vi "Test myTree.vi"() -> ()   [LabVIEW 2015, in "MyTreeAPI.lvclass"]
uses:
  MyTreeAPI.lvclass
  Menubar/Menu.lvclass
panel:
  in  "Tree":string(tree)
  out "ItemTag":string
  out "Node ID":string
  in  "Tag":string
  in  "OK Button":bool
  in  "stop":bool
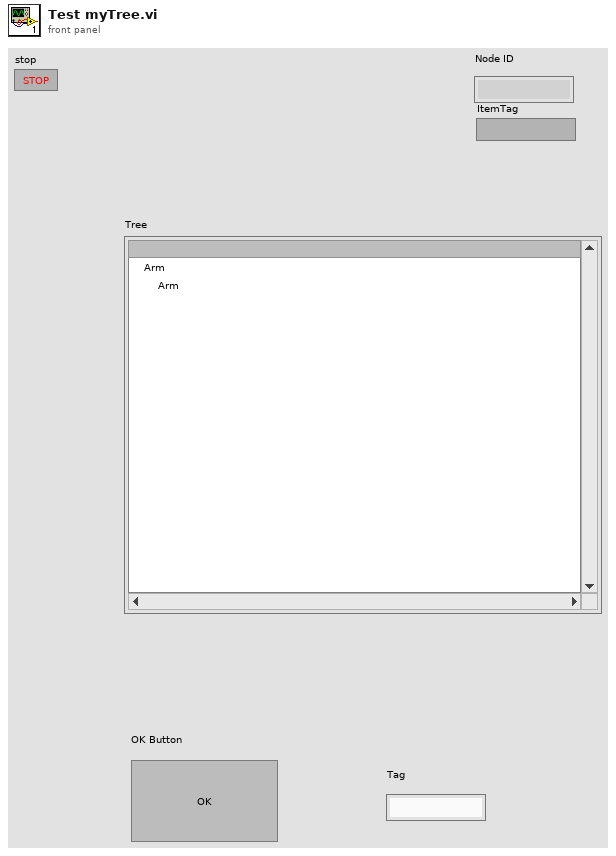
[diagram p1: front panel]
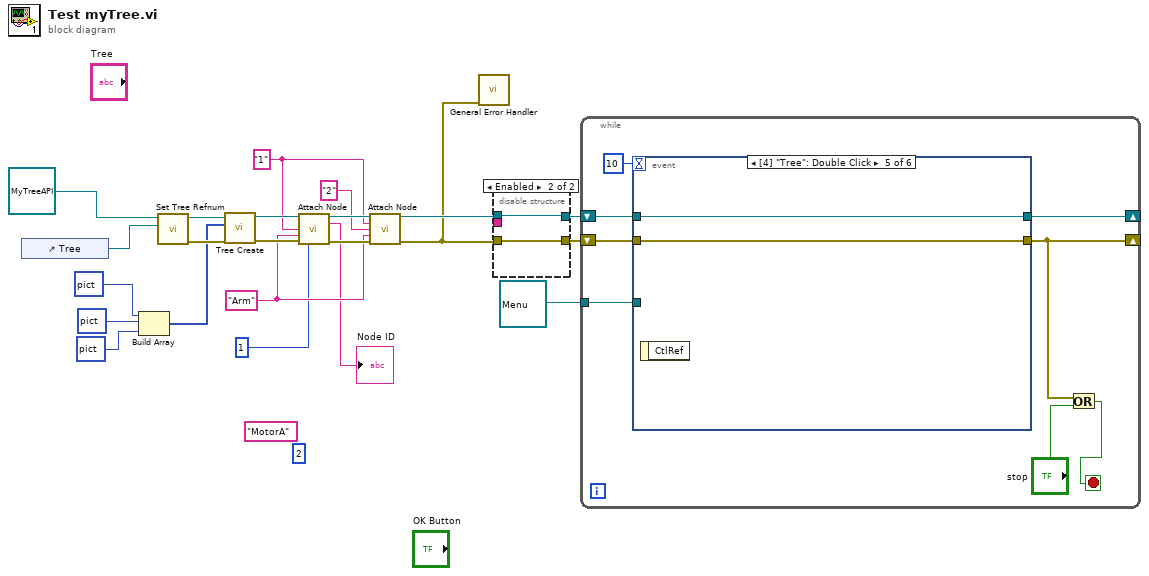
[diagram p0: block diagram]
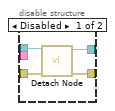
[diagram p2: hidden frame]
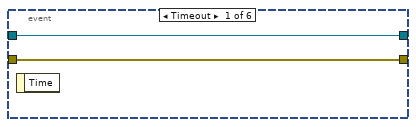
[diagram p3: hidden frame]
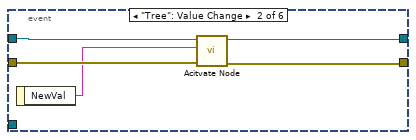
[diagram p4: hidden frame]
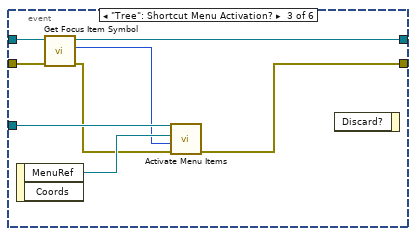
[diagram p5: hidden frame]
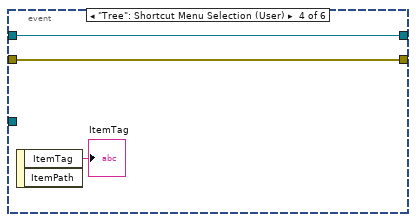
[diagram p6: hidden frame]
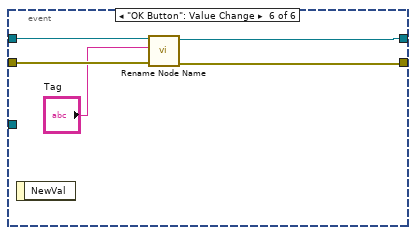
[diagram p7: hidden frame]
diagram:
  w8 = "1" ("Node ID")
  (unwired) 2 ("Symbol Index")
  (unwired) "MotorA" ("Node")
  w7 = "Arm" ("Tag")
  n1 = control-ref of="Tree"() -> (w1:refnum<vi>)
  n2 = Build Array(picture data[5B] ("2D Picture"), picture bytes[1570] ("2D Picture"), picture bytes[1570] ("2D Picture")) -> (w17:picture[])
  n3 = call "Set Tree Refnum.vi"("Tree"=w1, "TREE in"=refnum<class "MyTreeAPI.lvclass"> refnum) -> ("error out"=w20:errorcluster, "TREE out"=w21:refnum<class "MyTreeAPI.lvclass">)  [unwired: 8 in]
  n4 = call "Tree Create.vi"("error in (no error)"=w20, "Symbols"=w17, "TREE in"=w21) -> ("error out"=w15:errorcluster, "TREE out"=w16:refnum<class "MyTreeAPI.lvclass">)  [unwired: 7 in]
  n5 = call "Attach Node.vi"("TREE in"=w16, "Node ID"=w8, "Node Name"=w7, "error in (no error)"=w15, "Symbol Index"=1) -> ("TREE out"=w13:refnum<class "MyTreeAPI.lvclass">, "Node ID"=→"Node ID":string, "error out"=w12:errorcluster)  [unwired: 8 in]
  n6 = call "Attach Node.vi"("TREE in"=w13, "Parent Node"=w8, "Node ID"="2", "Node Name"=w7, "error in (no error)"=w12) -> ("TREE out"=w11:refnum<class "MyTreeAPI.lvclass">, "error out"=w3:errorcluster)  [unwired: 8 in, 1 out]
  n7 = call <vilib>:"General Error Handler.vi"("error in (no error)"=w3) -> ()  [unwired: 10 in, 5 out]
  n8 = disable-structure shown="Enabled" {
    disable-tunnel: w11 -> [w27 w29]
    disable-tunnel: w3 -> [w26 w28]
    disable-tunnel: [w25 w29] -> w10
    disable-tunnel: [w24 w28] -> w9
    disable-tunnel: _ -> [w23 _]
    frame Disabled {
      n9 = call "Detach Node.vi"("error in (no error)"=w26, "Node Name"=w23, "TREE in"=w27) -> ("error out"=w24:errorcluster, "TREE out"=w25:refnum<class "MyTreeAPI.lvclass">)  [unwired: 7 in]
    }
    frame Enabled {
    }
  }
  n10 = while {
    shift-right: [w34] -> _
    shift-left: w10 -> [w36]
    shift-right: [w33] -> _
    shift-left: w9 -> [w35]
    tunnel: refnum<class "Menu.lvclass"> refnum ("Menu") -> [w30]
    stop <- w31 stop-if-true
    n11 = event shown="[4] \"Tree\": Double Click" {
      selector: _ -> [_ _ _ _ _ _]
      dyn-events: _ -> [_ _ _ _ _ _]
      timeout: 10 -> [_ _ _ _ _ _]
      tunnel: w36 -> [w39 w44 w50 w54 w57 w62]
      tunnel: w35 -> [w38 w43 w49 w53 w56 w61]
      tunnel: [w39 w41 w47 w54 w57 w59] -> w34
      tunnel: [w38 w40 w45 w53 w56 w58] -> w33
      tunnel: w30 -> [_ _ w52 _ _ _]
      event Timeout {
        n12 = event-data() -> ()  [unwired: 1 in, 1 out]
      }
      event "Tree": Value Change {
        n13 = event-data() -> ("NewVal"=w42:string)  [unwired: 1 in]
        n14 = call "Acitvate Node.vi"("error in (no error)"=w43, "Active Node(\"\")"=w42, "TREE in"=w44) -> ("error out"=w40:errorcluster, "TREE out"=w41:refnum<class "MyTreeAPI.lvclass">)  [unwired: 7 in]
      }
      event "Tree": Shortcut Menu Activation? {
        n15 = event-data() -> ("MenuRef"=w51:refnum<k9>)  [unwired: 1 in, 1 out]
        n16 = call "Get Focus Item Symbol.vi"("error in (no error)"=w49, "MyTreeAPI in"=w50) -> ("error out"=w46:errorcluster, "Symbol"=w48:i32, "MyTreeAPI out"=w47:refnum<class "MyTreeAPI.lvclass">)  [unwired: 7 in]
        n17 = call-dynamic "Activate Menu Items.vi"("error in (no error)"=w46, "State(0)"=w48, "MenuRefnum"=w51, "Menu in"=w52) -> ("error out"=w45:errorcluster)  [unwired: 6 in, 1 out]
        n18 = event-data() -> ()  [unwired: 2 in, 1 out]
      }
      event "Tree": Shortcut Menu Selection (User) {
        n19 = event-data() -> ("ItemTag"=→"ItemTag":string)  [unwired: 1 in, 1 out]
      }
      event "Tree": Double Click {
        n20 = event-data() -> ()  [unwired: 1 in, 1 out]
      }
      event "OK Button": Value Change {
        n21 = event-data() -> ()  [unwired: 1 in, 1 out]
        n22 = call "Rename Node Name.vi"("error in (no error)"=w61, "Node Tag"="Tag", "TREE in"=w62) -> ("error out"=w58:errorcluster, "TREE out"=w59:refnum<class "MyTreeAPI.lvclass">)  [unwired: 7 in]
      }
    }
    n23 = Or(x=w33, y="stop") -> (x .or. y?=w31:bool)
  }
